vi "main_getPh.vi"(10 "Running?":refnum<vi>, 11 "PH":refnum<vi>) -> ()   [LabVIEW 2019]
uses:
  lib/libFileFunctions/libFileFunctions.lvlib
  lib/libSimulationControl/libSimulationControl.lvlib
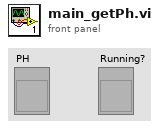
[diagram p1: front panel]
types:
  T1 = enum8{"Enabled", "Disabled", "Disabled and Grayed Out"}
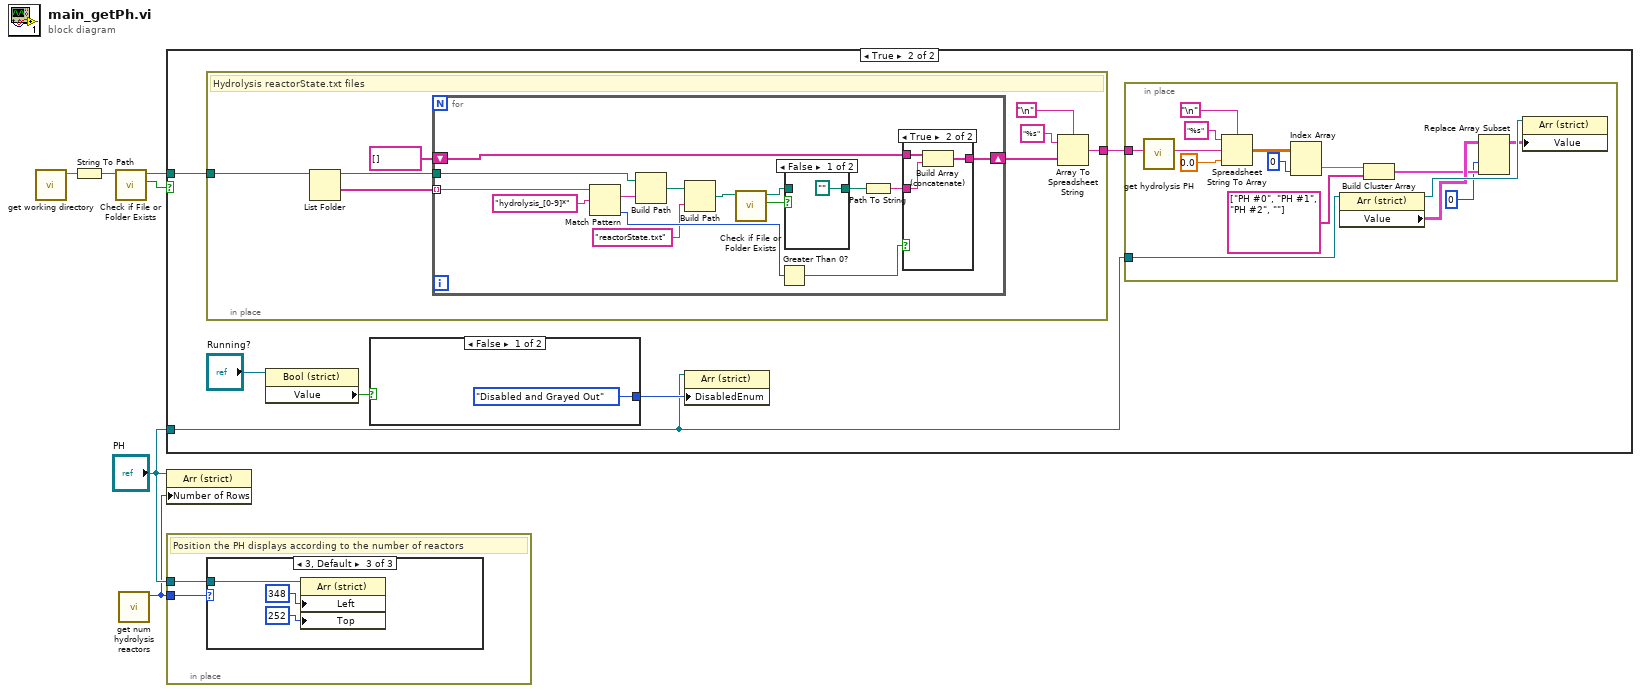
[diagram p0: block diagram]
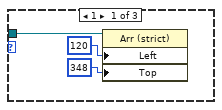
[diagram p2: hidden frame]
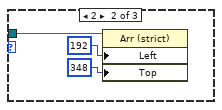
[diagram p3: hidden frame]
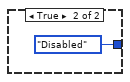
[diagram p5: hidden frame]
diagram:
  n1 = call "get working directory.vi"() -> ("function return"=w6:string)  [unwired: 10 in, 1 out]
  n2 = String To Path(string=w6) -> (path=w5:path)
  n3 = call <vilib>:"Check if File or Folder Exists.vi"("path"=w5) -> ("file or folder exists?"=w3:bool, "dup path"=w4:path)  [unwired: 8 in, 1 out]
  n4 = call "get num hydrolysis reactors.vi"() -> ("function return"=w1:i32)  [unwired: 10 in, 1 out]
  n5 = case shown="True" w3 {
    tunnel: "PH" -> [_ w7]
    tunnel: w4 -> [_ w12]
    frame False {
    }
    frame True {
      # "Set PH display value"
      n6 = in-place {
        in-place-border: w12 -> [w31]
        in-place-border: [w30] -> w8
        # "Hydrolysis reactorState.txt files"
        n7 = List Folder(path=w31) -> (path out=w35:path, folder names=w37:string[])  [unwired: 3 in, 2 out]
        n8 = for {
          tunnel: w37 -> [w47] mode=indexing
          shift-right: [w48] -> w34
          shift-left: string[] [] -> [w49]
          tunnel: w35 -> [w46]
          n9 = Match Pattern(string=w47, regular expression="hydrolysis_[0-9]*") -> (match substring=w45:string, offset past match=w50:i32)  [unwired: 1 in, 2 out]
          n10 = Build Path(base path=w46, name or relative path=w45) -> (appended path=w44:path)
          n11 = Build Path(base path=w44, name or relative path="reactorState.txt") -> (appended path=w41:path)
          n12 = call <vilib>:"Check if File or Folder Exists.vi"("path"=w41) -> ("file or folder exists?"=w40:bool, "dup path"=w39:path)  [unwired: 8 in, 1 out]
          n13 = Greater Than 0?(x=w50) -> (x > 0?=w51:bool)
          n14 = case shown="False" w40 {
            tunnel: [path "" w54] -> w38
            tunnel: w39 -> [_ w54]
            frame False {
            }
            frame True {
            }
          }
          n15 = Path To String(path=w38) -> (string=w42:string)
          n16 = case shown="True" w51 {
            tunnel: [w55 w58] -> w48
            tunnel: w49 -> [w55 w57]
            tunnel: w42 -> [_ w56]
            frame False {
            }
            frame True {
              n17 = Build Array (concatenate)(w57, w56) -> (w58:string[])
            }
          }
        }
        n18 = Array To Spreadsheet String(delimiter (Tab)="\n", array=w34, 3:"%s" ("format string")) -> (spreadsheet string=w30:string)
      }
      n19 = property class="Bool (strict)"(reference="Running?") -> ("Value"=w9:bool)  [unwired: 1 in, 2 out]
      n20 = case shown="False" w9 {
        tunnel: [T1."Disabled and Grayed Out" ("Disabled") T1."Disabled" ("Disabled")] -> w11
        frame False {
        }
        frame True {
        }
      }
      n21 = property on="Property Node" class="Arr (strict)"(reference=w7, "DisabledEnum"=w11) -> ()  [unwired: 1 in, 2 out]
      n22 = in-place {
        in-place-border: w7 -> [w27]
        in-place-border: w8 -> [w26]
        n23 = call "get hydrolysis PH.vi"("reactor_state_files"=w26) -> ("ph_string"=w23:string)  [unwired: 9 in, 1 out]
        n24 = Spreadsheet String To Array(delimiter (Tab)="\n", format string="%s", spreadsheet string=w23, array type (2D Dbl)=0.0) -> (array=w19:dbl[][])
        n25 = Index Array(array=w19, index (col)=0 ("disabled index (col)")) -> (element=w18:dbl[])  [unwired: 1 in]
        n26 = property on="Property Node" class="Arr (strict)"(reference=w27) -> (reference out=w25:refnum<vi>, "Value"=w16:cluster{"Meter":dbl, "String":string}[][])  [unwired: 1 in, 1 out]
        n27 = Build Cluster Array(w18, string[] ["PH #0", "PH #1", "PH #2", ""] ("Set Names")) -> (w15:cluster{dbl, "String":string}[])
        n28 = Replace Array Subset(array=w16, new element=w15, index (col)=0 ("index (row)")) -> (w14:cluster{"Meter":dbl, "String":string}[][])  [unwired: 1 in]
        n29 = property on="Property Node" class="Arr (strict)"(reference=w25, "Value"=w14) -> ()  [unwired: 1 in, 2 out]
      }
    }
  }
  n30 = property class="Arr (strict)"(reference="PH", "Number of Rows"=w1) -> ()  [unwired: 1 in, 2 out]
  n31 = in-place {
    in-place-border: w1 -> [w60]
    in-place-border: "PH" -> [w59]
    # "Position the PH displays according to the number of reactors"
    n32 = case shown="3, Default" w60 {
      tunnel: w59 -> [w63 w66 w69]
      frame 1 {
        n33 = property class="Arr (strict)"(reference=w63, "Left"=120 ("Position:Left"), "Top"=348 ("Position:Top")) -> ()  [unwired: 1 in, 2 out]
      }
      frame 2 {
        n34 = property class="Arr (strict)"(reference=w66, "Left"=192 ("Position:Left"), "Top"=348 ("Position:Top")) -> ()  [unwired: 1 in, 2 out]
      }
      frame 3, Default {
        n35 = property class="Arr (strict)"(reference=w69, "Left"=348 ("Position:Left"), "Top"=252 ("Position:Top")) -> ()  [unwired: 1 in, 2 out]
      }
    }
  }
